vi "Configure Modulation (Amplitude).vi"(0 "VISA resource name":refnum<visa-resource-name>, 1 "Enable Amplitude Modulation (T: Enable)":bool=TRUE, 5 "Channel (0: Channel 1)":u16(ring) items=["Channel 1", "Channel 2"], 7 "AM Source (0: Internal)":u16(ring) items=["Internal", "External"], 9 "Modulation Waveform (0: Sine)":u16(ring) items=["Sine", "Square", "Triangle", "Ramp", "Down Ramp", "Noise", "User 1", "User 2", "User 3", "User 4", "Edit Memory"], 11 "error in (no error)":errorcluster, 12 "Modulation Frequency (1000 Hz)":dbl=1000.0, 13 "Modulation Depth (0 %)":dbl) -> (4 "VISA resource name out":refnum<visa-resource-name>, 15 "error out":errorcluster)   [LabVIEW 2013, in "AWG.lvlib" / "Tektronix AFG 3000 Series.lvlib"]
doc: "Configures and enables amplitude modulation (AM). In AM, the amplitude of the carrier is varied by the amplitude of the modulating waveform."
uses:
  Tektronix AFG 3000 Series.lvlib
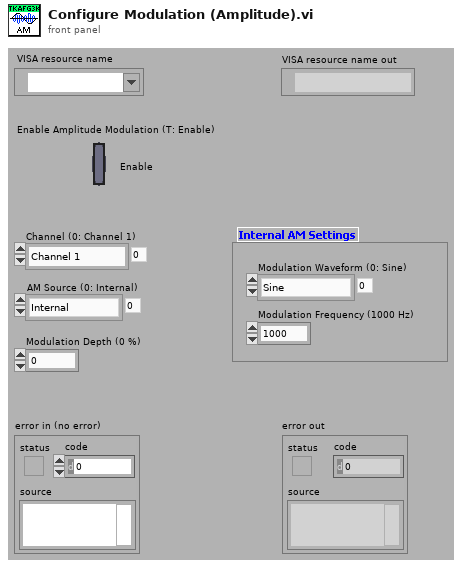
[diagram p1: front panel]
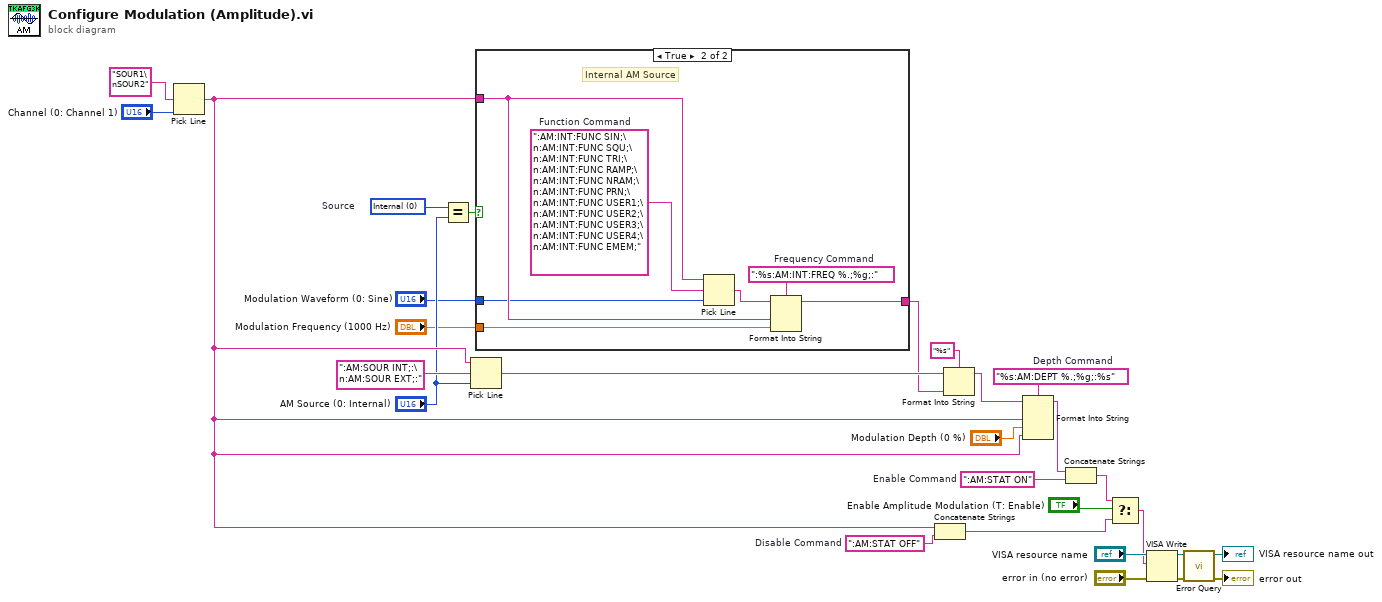
[diagram p0: block diagram]
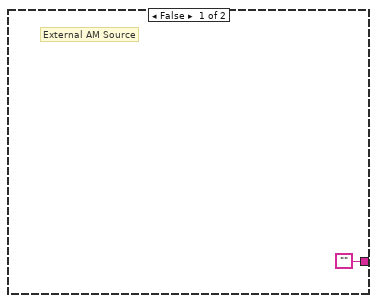
[diagram p2: hidden frame]
diagram:
  w18 = ":AM:STAT ON"  # Enable Command
  w20 = "%s:AM:DEPT %.;%g;:%s"  # Depth Command
  w4 = u16 0 items=["Internal", "External"]  # Source
  w12 = ":AM:STAT OFF"  # Disable Command
  n1 = Pick Line(multi-line string="SOUR1\nSOUR2" ("string (\"\")"), line index="Channel (0: Channel 1)") -> (output string=w10:string)  [unwired: 1 in]
  n2 = Equal?(x=w4, y="AM Source (0: Internal)") -> (x = y?=w9:bool)
  n3 = Pick Line(string ("")=w10, multi-line string=":AM:SOUR INT;:\n:AM:SOUR EXT;:" ("Source Command"), line index="AM Source (0: Internal)") -> (output string=w7:string)
  n4 = case shown="True" w9 {
    tunnel: w10 -> [_ w32]
    tunnel: ["" w33] -> w6
    tunnel: "Modulation Waveform (0: Sine)" -> [_ w31]
    tunnel: "Modulation Frequency (1000 Hz)" -> [_ w30]
    frame False {
      # "External AM Source"
    }
    frame True {
      w35 = ":%s:AM:INT:FREQ %.;%g;:"  # Frequency Command
      w36 = ":AM:INT:FUNC SIN;\n:AM:INT:FUNC SQU;\n:AM:INT:FUNC TRI;\n:AM:INT:FUNC RAMP;\n:AM:INT:FUNC NRAM;\n:AM:INT:FUNC PRN;\n:AM:INT:FUNC USER1;\n:AM:INT:FUNC USER2;\n:AM:INT:FUNC USER3;\n:AM:INT:FUNC USER4;\n:AM:INT:FUNC EMEM;"  # Function Command
      # "Internal AM Source"
      n5 = Pick Line(string ("")=w32, multi-line string=w36, line index=w31) -> (output string=w34:string)
      n6 = Format Into String(format string=w35, initial string=w34, w32, w30) -> (resulting string=w33:string)  [unwired: 1 in, 1 out]
    }
  }
  n7 = Concatenate Strings(w10, w12) -> (w11:string)
  n8 = Format Into String(format string="%s", initial string=w7, w6) -> (resulting string=w5:string)  [unwired: 1 in, 1 out]
  n9 = Format Into String(format string=w20, initial string=w5, w10, "Modulation Depth (0 %)", w10) -> (resulting string=w19:string)  [unwired: 1 in, 1 out]
  n10 = Concatenate Strings(w19, w18) -> (w14:string)
  n11 = Select(t=w14, s="Enable Amplitude Modulation (T: Enable)", f=w11) -> (s? t:f=w15:string)
  n12 = VISA Write(VISA resource name="VISA resource name", write buffer=w15, error in (no error)="error in (no error)") -> (VISA resource name out=w24:refnum<visa-resource-name>, error out=w23:errorcluster)  [unwired: 1 out]
  n13 = call "Error Query.vi"("error in (no error)"=w23, "VISA resource name"=w24) -> ("error out"=→"error out":errorcluster, "VISA resource name out"=→"VISA resource name out":refnum<visa-resource-name>)  [unwired: 6 in, 2 out]
